vi "get next modbus address.vi"(0 "Modbus Slave configuration in":refnum<class "Modbus Module configuration.lvclass">, 5 "modbus channels":refnum<class "Modbus Module Channel.lvclass">[](array[class]), 7 "modbus address":T1(array[cluster]), 9 "channel indices":i32[](array[numeric]), 11 "error in":errorcluster) -> (4 "Modbus Slave configuration out":refnum<class "Modbus Module configuration.lvclass">, 8 "modbus address out":T1(array[cluster]), 15 "error out":errorcluster)   [LabVIEW 2015, in "Modbus Module configuration.lvclass"]
uses:
  Modbus Module configuration.lvclass
  module channel/Modbus Module Channel.lvclass
  module channel/Modbus Module Channel.lvclass/Modbus Module Channel.ctl
  <vilib>/NI/Tag Bus/tag/tag descriptor.lvclass/tag descriptor.ctl
  module channel/Read modbus type.vi
  <vilib>/NI/Tag Bus/tag/read data type.vi
  module channel/Read subindex (bool).vi
  module channel/Write starting address.vi
  module channel/Write subindex (bool).vi
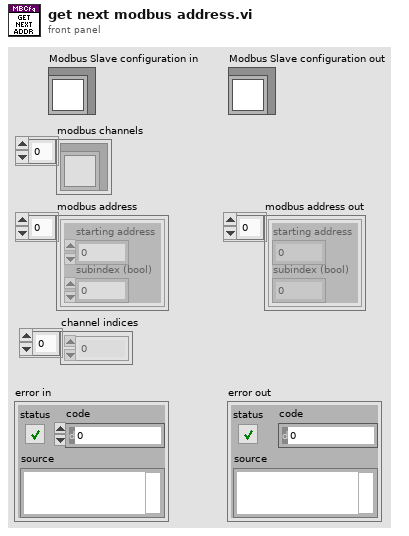
[diagram p1: front panel]
types:
  T1 = cluster{"starting address":u16, "subindex (bool)":i32}[]
  T2 = typedef "Modbus Module Channel.lvclass/data bank type.ctl" = enum16{"Coils", "Discrete Inputs", "Input Registers", "Holding Registers"}
  T3 = typedef "tag bus.lvlib/tag descriptor.lvclass/Data Type.ctl" = enum16{"Double", "Single", "I64", "I32", "I16", "I8", "U64", "U32", "U16", "U8", "Boolean", "String", "Array of Double", "Array of Single", "Array of I64", "Array of I32", "Array of I16", "Array of I8", "Array of U64", "Array of U32", "Array of U16", "Array of U8", "Array of Boolean", "Array of String"}
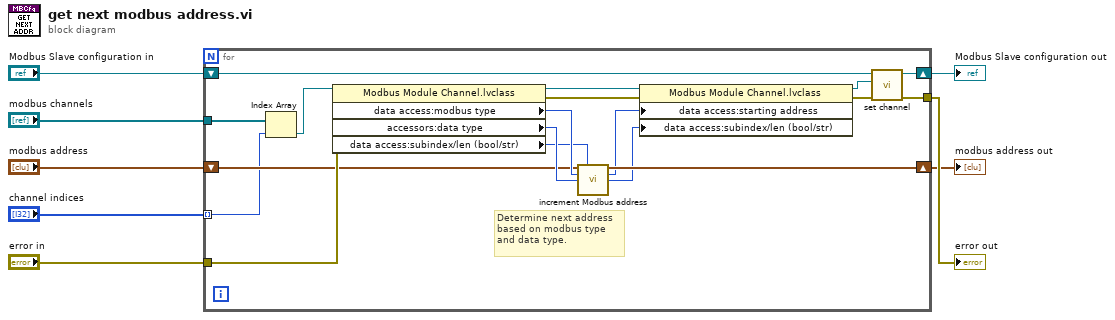
[diagram p0: block diagram]
diagram:
  n1 = for {
    tunnel: "modbus channels" -> [w11]
    shift-right: [w17] -> w1
    shift-left: "modbus address" -> [w18]
    shift-right: [w25] -> w5
    shift-left: "Modbus Slave configuration in" -> [w13]
    tunnel: "error in" -> [w24]
    tunnel: [w21] -> w6
    tunnel: "channel indices" -> [w12] mode=indexing
    # "Determine next address \nbased on modbus type \nand data type."
    n2 = Index Array(array=w11, index=w12) -> (element=w10:refnum<class "Modbus Module Channel.lvclass">)
    n3 = property class="Modbus Module Channel.lvclass"(reference=w10, error in=w24) -> (reference out=w14:refnum<class "Modbus Module Channel.lvclass">, error out=w23:errorcluster, "data access:modbus type"=w19:T2, "accessors:data type"=w20:T3, "data access:subindex/len (bool/str)"=w9:i32)
    n4 = call "increment Modbus address.vi"("available addresses"=w18, "string length"=w9, "modbus type"=w19, "data type"=w20) -> ("available addresses out"=w17:T1, "starting address"=w16:u16, "subindex (bool)"=w15:i32)  [unwired: 9 in]
    n5 = property class="Modbus Module Channel.lvclass"(reference=w14, error in=w23, "data access:starting address"=w16, "data access:subindex/len (bool/str)"=w15) -> (reference out=w26:refnum<class "Modbus Module Channel.lvclass">, error out=w22:errorcluster)
    n6 = call "set channel.vi"("error in"=w22, "Modbus Module Channel.lvclass"=w26, "Modbus Slave configuration in"=w13) -> ("error out"=w21:errorcluster, "Modbus Slave configuration out"=w25:refnum<class "Modbus Module configuration.lvclass">)  [unwired: 7 in]
  }
  "error out" <- w6
  "Modbus Slave configuration out" <- w5
  "modbus address out" <- w1
